vi "Decode.vi"(8 "error in (no error)":errorcluster, 10 "Clear Raw Data":bool caption="Clear Raw Data(False)", 11 "Raw Data":string) -> (0 "error out":errorcluster, 1 "Success":bool, 2 "Sequence No":string, 3 "Data":string)   [LabVIEW 2019]
uses:
  Step.ctl
  Sign.ctl
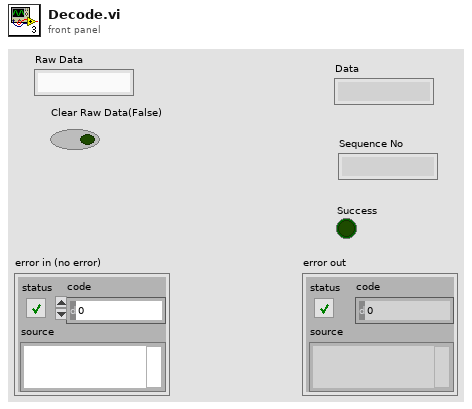
[diagram p1: front panel]
types:
  T1 = typedef "Step.ctl" = enum16{"找A帧头", "找A序号", "找A数据", "找B帧头", "找B序号", "找B数据"}
  T2 = typedef "Sign.ctl" = i32
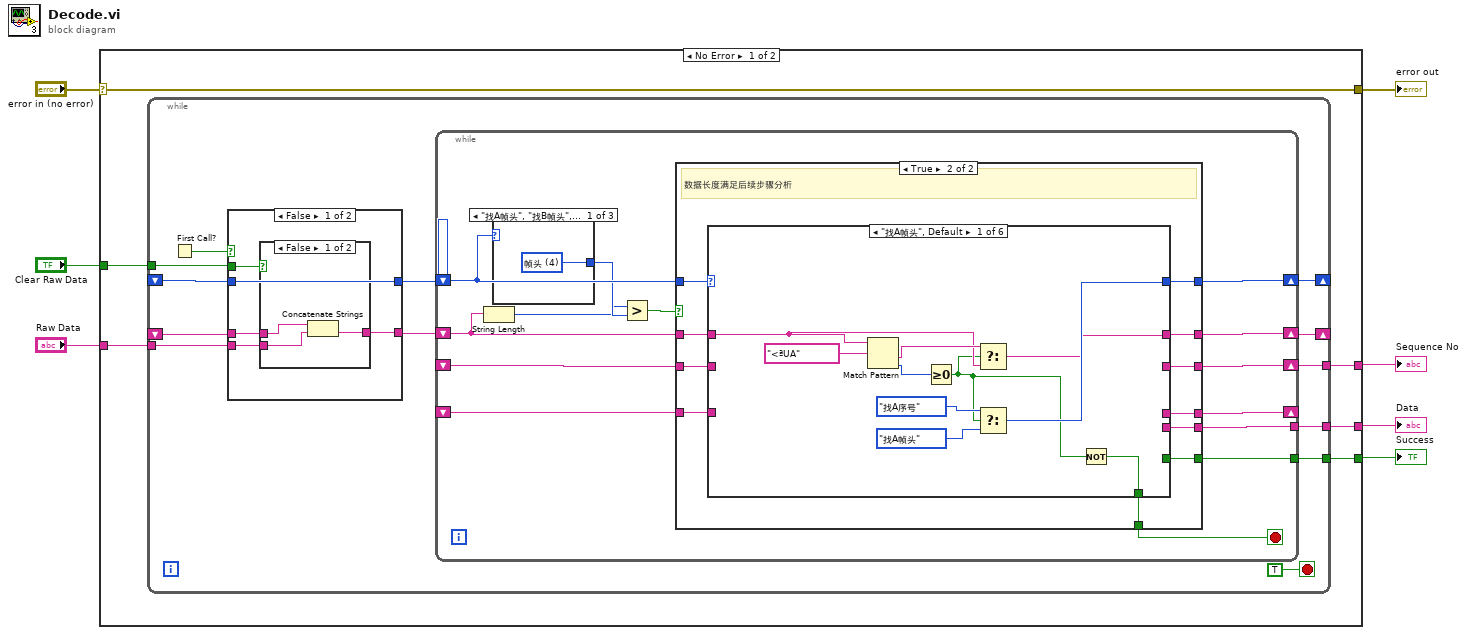
[diagram p0: block diagram]
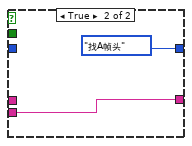
[diagram p3: hidden frame]
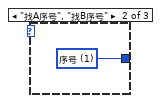
[diagram p4: hidden frame]
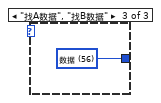
[diagram p5: hidden frame]
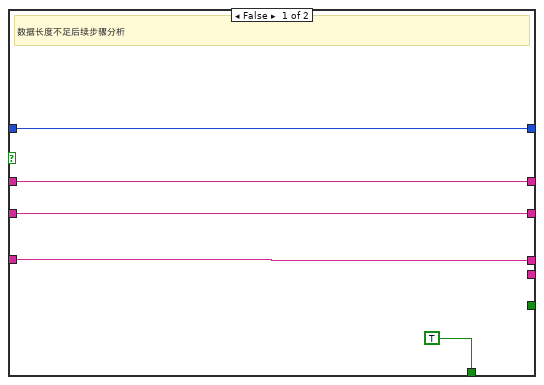
[diagram p6: hidden frame]
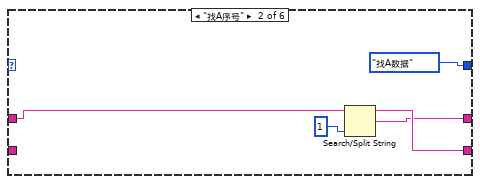
[diagram p7: hidden frame]
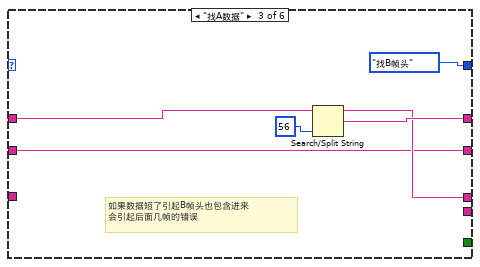
[diagram p8: hidden frame]
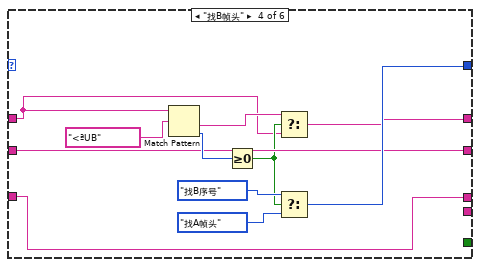
[diagram p9: hidden frame]
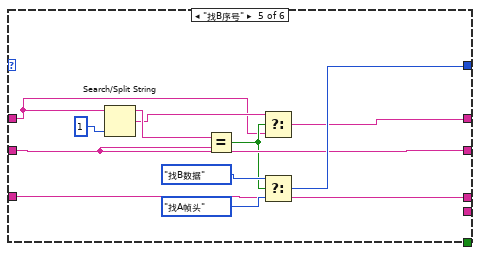
[diagram p10: hidden frame]
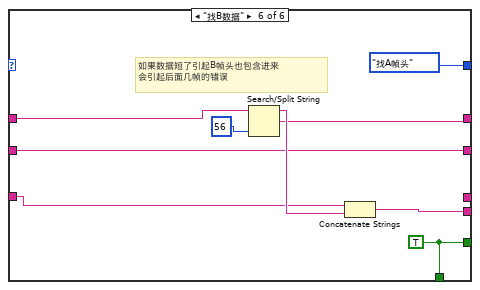
[diagram p11: hidden frame]
diagram:
  n1 = case shown="No Error" "error in (no error)" {
    selector: "error in (no error)" -> [w8 w123]
    tunnel: "Raw Data" -> [w13 _]
    tunnel: "Clear Raw Data" -> [w12 _]
    tunnel: [w11 _] -> w5
    tunnel: [w10 _] -> w4
    tunnel: [w9 _] -> w3
    tunnel: [w8 w123] -> w1
    frame No Error {
      n2 = while {
        tunnel: [w25] -> w9
        shift-right: [w26] -> _
        shift-left: _ -> [w15]
        tunnel: [w24] -> w10
        tunnel: [w23] -> w11
        tunnel: w13 -> [w16]
        tunnel: w12 -> [w17]
        shift-right: [w18] -> _
        shift-left: _ -> [w19]
        stop <- TRUE stop-if-true
        n3 = First Call?() -> (First Call?: T/F=w21:bool)
        n4 = case shown="False" w21 {
          tunnel: [w31 Step."找A帧头"] -> w20
          tunnel: w19 -> [w31 _]
          tunnel: w17 -> [w30 _]
          tunnel: w16 -> [w29 w36]
          tunnel: w15 -> [w28 _]
          tunnel: [w27 w36] -> w14
          frame False {
            n5 = case shown="False" w30 {
              tunnel: [w34 w35] -> w27
              tunnel: w29 -> [w33 w35]
              tunnel: w28 -> [w32 _]
              frame False {
                n6 = Concatenate Strings(w32, w33) -> (w34:string)
              }
              frame True {
              }
            }
          }
          frame True {
          }
        }
        n7 = while {
          shift-right: [w50] -> w18
          shift-left: w20 -> [w48]
          shift-right: [w49] -> w26
          shift-left: w14 -> [w51]
          shift-right: [w43] -> w25
          shift-left: _ -> [w42]
          shift-right: [w41] -> _
          shift-left: _ -> [w40]
          tunnel: [w39] -> w23
          tunnel: [w38] -> w24
          stop <- w44 stop-if-true
          n8 = String Length(string=w51) -> (length=w46:i32)
          n9 = case shown="\"找A帧头\", \"找B帧头\", Default" w48 {
            tunnel: [w52 w53 w54] -> w47
            frame "找A帧头", "找B帧头", Default {
              w52 = T2 4 items=["帧头"=4, "序号"=1, "数据"=56]
            }
            frame "找A序号", "找B序号" {
              w53 = T2 1 items=["帧头"=4, "序号"=1, "数据"=56]
            }
            frame "找A数据", "找B数据" {
              w54 = T2 56 items=["帧头"=4, "序号"=1, "数据"=56]
            }
          }
          n10 = Greater?(x=w46, y=w47) -> (0:w45:bool)
          n11 = case shown="True" w45 {
            tunnel: w48 -> [w58 w70]
            tunnel: w51 -> [w59 w69]
            tunnel: [w58 w68] -> w50
            tunnel: [w59 w67] -> w49
            tunnel: [TRUE w64] -> w44
            tunnel: [w56 w66] -> w43
            tunnel: w42 -> [w56 w65]
            tunnel: [w55 w63] -> w41
            tunnel: w40 -> [w55 w62]
            tunnel: [_ w61] -> w39
            tunnel: [_ w60] -> w38
            frame False {
              # "数据长度不足后续步骤分析"
            }
            frame True {
              # "数据长度满足后续步骤分析"
              n12 = case shown="\"找A帧头\", Default" w70 {
                tunnel: w69 -> [w73 w84 w87 w93 w105 w121]
                tunnel: [w77 Step."找A数据" Step."找B帧头" ("f") w99 w110 Step."找A帧头" ("f")] -> w68
                tunnel: [w75 w82 w90 w94 w104 w114] -> w67
                tunnel: [_ w83 w86 w98 w109 w115] -> w66
                tunnel: w65 -> [_ _ w86 w98 w109 w115]
                tunnel: [w72 _ _ _ _ w117] -> w64
                tunnel: [_ _ w89 w92 w103 _] -> w63
                tunnel: w62 -> [_ _ _ w92 w103 w119]
                tunnel: [_ _ _ _ _ w117] -> w61
                tunnel: [_ _ _ _ _ w116] -> w60
                frame "找A帧头", Default {
                  n13 = Match Pattern(string=w73, regular expression="<ªUA") -> (after substring=w76:string, offset past match=w79:i32)  [unwired: 1 in, 2 out]
                  n14 = Greater Or Equal To 0?(x=w79) -> (x >= 0?=w71:bool)
                  n15 = Select(t=w76, s=w71, f=w73) -> (s? t:f=w75:string)
                  n16 = Select(t=Step."找A序号", s=w71, f=Step."找A帧头") -> (s? t:f=w77:T1)
                  n17 = Not(x=w71) -> (.not. x?=w72:bool)
                }
                frame "找A序号" {
                  n18 = Search/Split String(string=w84, offset (0)=1) -> (substring before match=w83:string, match + rest of string=w82:string)  [unwired: 1 in, 1 out]
                }
                frame "找A数据" {
                  # "如果数据短了引起B帧头也包含进来\n会引起后面几帧的错误"
                  n19 = Search/Split String(string=w87, offset (0)=56) -> (substring before match=w89:string, match + rest of string=w90:string)  [unwired: 1 in, 1 out]
                }
                frame "找B帧头" {
                  n20 = Match Pattern(string=w93, regular expression="<ªUB") -> (after substring=w95:string, offset past match=w102:i32)  [unwired: 1 in, 2 out]
                  n21 = Greater Or Equal To 0?(x=w102) -> (x >= 0?=w96:bool)
                  n22 = Select(t=w95, s=w96, f=w93) -> (s? t:f=w94:string)
                  n23 = Select(t=Step."找B序号", s=w96, f=Step."找A帧头") -> (s? t:f=w99:T1)
                }
                frame "找B序号" {
                  n24 = Search/Split String(string=w105, offset (0)=1) -> (substring before match=w112:string, match + rest of string=w107:string)  [unwired: 1 in, 1 out]
                  n25 = Equal?(x=w112, y=w109) -> (x = y?=w106:bool)
                  n26 = Select(t=w107, s=w106, f=w105) -> (s? t:f=w104:string)
                  n27 = Select(t=Step."找B数据", s=w106, f=Step."找A帧头") -> (s? t:f=w110:T1)
                }
                frame "找B数据" {
                  w117 = TRUE
                  # "如果数据短了引起B帧头也包含进来\n会引起后面几帧的错误"
                  n28 = Search/Split String(string=w121, offset (0)=56) -> (substring before match=w120:string, match + rest of string=w114:string)  [unwired: 1 in, 1 out]
                  n29 = Concatenate Strings(w119, w120) -> (w116:string)
                }
              }
            }
          }
        }
      }
    }
    frame Error {
    }
  }
  "error out" <- w1
  "Sequence No" <- w3
  "Data" <- w4
  "Success" <- w5
